vi "Read Measurements.vi"(8 "error in (no error)":errorcluster, 11 "Scope in":refnum<class "Scope Instrument.lvclass">) -> (0 "error out":errorcluster, 1 "Waveforms":waveform(dbl)[](array[waveform]), 2 "Measurements":T1[](array[typedef]) {"Lower limit" format="%#_4p"; "Upper limit" format="%#_4p"}, 3 "Scope out":refnum<class "Scope Instrument.lvclass">)   [LabVIEW 2025, in "Scope.lvlib" / "Scope Instrument.lvclass"]
uses:
  Scope Instrument.lvclass
  Users/Public/Documents/Sandia National Labs/TSS Plugin/Abstract Engine.lvlibp/Abstract Instrument/Channel.ctl
  Scope Instrument.lvclass/Scope Instrument.ctl
  Users/Public/Documents/Sandia National Labs/TSS Plugin/Abstract Engine.lvlibp/Abstract Instrument/Abstract Instrument.lvclass
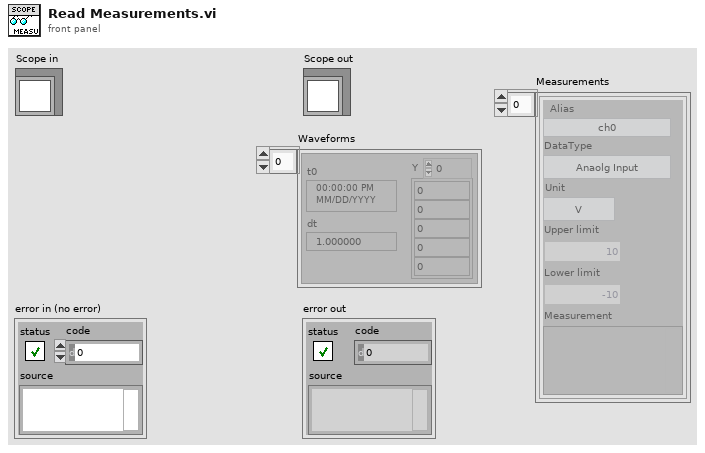
[diagram p1: front panel]
types:
  T1 = typedef "Abstract Engine.lvlibp/Abstract Instrument.lvclass/Channel.ctl" = cluster{"Alias":string, "DataType":enum16{"Anaolg Input", "Waveform"}, "Unit":enum16{"---", "V", "A", "Ohm", "Hz", "uF", "degC", "deg"}, "Upper limit":dbl, "Lower limit":dbl, "Measurement":variant}
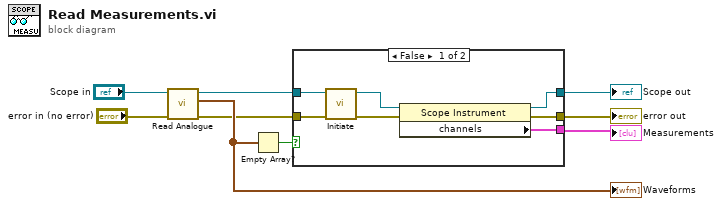
[diagram p0: block diagram]
diagram:
  n1 = call-dynamic "Read Analogue.vi"("error in (no error)"="error in (no error)", "Analog Input in"="Scope in") -> ("error out"=w4:errorcluster, "Waveforms"=w7:waveform(dbl)[], "Analog Input out"=w5:refnum<class "Scope Instrument.lvclass">)  [unwired: 7 in]
  "Waveforms" <- w7
  n2 = Empty Array?(array=w7) -> (empty?=w6:bool)
  n3 = case shown="False" w6 {
    tunnel: w5 -> [w16 w18]
    tunnel: w4 -> [w15 w17]
    tunnel: [w12 w17] -> w3
    tunnel: [w11 w18] -> w1
    tunnel: [w10 _] -> w2
    frame False {
      n4 = call-dynamic "Initiate.vi"("error in (no error)"=w15, "Scope Instrument in"=w16) -> ("error out"=w13:errorcluster, "Scope Instrument out"=w14:refnum<class "Scope Instrument.lvclass">)  [unwired: 8 in]
      n5 = property class="Scope Instrument"(reference=w14, error in=w13) -> (reference out=w11:refnum<class "Scope Instrument.lvclass">, error out=w12:errorcluster, "channels"=w10:T1[])
    }
    frame True {
    }
  }
  "error out" <- w3
  "Scope out" <- w1
  "Measurements" <- w2
